vi "Read Full Output.vi"(6 "maximal byte count (-1)":i32=-1, 7 "timeout [ms]":u32=10, 8 "error in":errorcluster, 11 "GOLPI ref. in":T1={"pipe handle"={"lv_proc.dll file path"=path "", "process instance handle"=[], "debug mode"=FALSE, "debug data"=[]}, "fast read timeout [ms]"=500, "fast read settle time [ms]"=10, "fast read to multiple [ms]"=1, "max elements per input line"=100, "slow read timeout [ms]"=5000, "stdin double format specifier"="%_16e", "max elements per stdout output column"=100, "console mode bitstream"=FALSE, "bitstream first read timeout [ms]"=1000, "bitstream read timeout [ms]"=50, "struct transfer possible"=FALSE, "matlab mode"=FALSE}) -> (0 "error out":errorcluster, 2 "read buffer":string, 3 "GOLPI ref. out":T1={"pipe handle"={"lv_proc.dll file path"=path "", "process instance handle"=[], "debug mode"=FALSE, "debug data"=[]}, "fast read timeout [ms]"=500, "fast read settle time [ms]"=10, "fast read to multiple [ms]"=1, "max elements per input line"=100, "slow read timeout [ms]"=5000, "stdin double format specifier"="%_16e", "max elements per stdout output column"=100, "console mode bitstream"=FALSE, "bitstream first read timeout [ms]"=1000, "bitstream read timeout [ms]"=50, "struct transfer possible"=FALSE, "matlab mode"=FALSE}, 5 "bytes remaining":i32)   [LabVIEW 2020, in "GOLPI library.lvlib"]
doc: "Reads full output of GNU Octave in stdout pipe.\nIf timeout is exceeded (i.e. buffer contains too many characters), returns only part of buffer and returns number of bytes remaining in the stdout (if any).\nReading also stops if maximal byte count terminal is set to natural nonzero value and number of red bytes reaches this limit.\n\n---\nGOLPI works only with lv_proc.dll library, which is part of vipm package or should be delivered together with packed library. Placement of this dll is selected in terminal of Start GNU Octave.vi."
uses:
  GOLPI library.lvlib
  GOLPI reference Type Def.ctl
  Pipe Handle.ctl
  Custom Error Codes Enum Type Def.vi
  LV Process library.lvlib
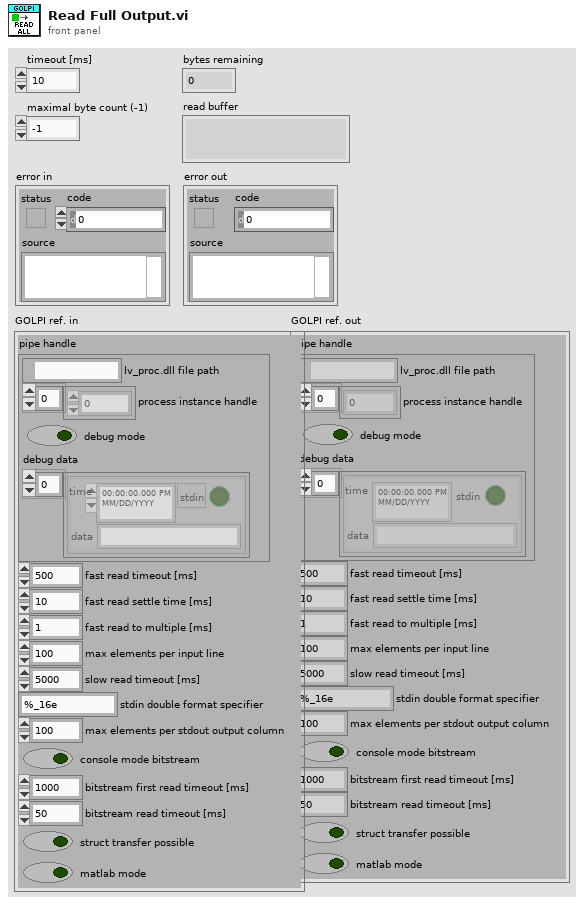
[diagram p1: front panel]
types:
  T1 = typedef "GOLPI library.lvlib/GOLPI reference Type Def.ctl" = cluster{"pipe handle":T2, "fast read timeout [ms]":u32, "fast read settle time [ms]":u32, "fast read to multiple [ms]":u32, "max elements per input line":u32, "slow read timeout [ms]":u32, "stdin double format specifier":string, "max elements per stdout output column":u32, "console mode bitstream":bool, "bitstream first read timeout [ms]":u32, "bitstream read timeout [ms]":u32, "struct transfer possible":bool, "matlab mode":bool}
  T2 = typedef "LV Process library.lvlib/Pipe Handle.ctl" = cluster{"lv_proc.dll file path":path, "process instance handle":u32[], "debug mode":bool, "debug data":cluster{"time":timestamp, "stdin":bool, "data":string}[]}
  T3 = typedef "GOLPI library.lvlib/Custom Error Codes Enum Type Def.vi" = enum16{"no error", "00 working directory PAR1 missing", "01 octave binary PAR1 missing", "02 octave report error PAR1", "03 empty output last cmd PAR1", "04 missing temporary file PAR1", "05 pwd PAR 1 not exist", "06 oct package not installed", "07 octave default binary missing", "10 var PAR1 not string, vect", "11 var PAR1 not num, scal, ~compl", "12 var PAR1 not num, scal, compl", "13 var PAR1 not num, vect, ~compl", "14 var PAR1 not num, vect, compl", "15 var PAR1 not num, mat, ~compl", "16 var PAR1 not num, mat, ~compl", "30 read timeout", "60 bitstream transport failed", "61 bitstream decode error PAR1", "62 bitstream cannot be set", "70 struct transfer not possible", "80 struct: cluster elem. PAR1 not implem.", "81 struct: structure field PAR1 not implem.", "82 struct: size mismatch of PAR1", "83 struct: type mismatch of PAR1", "98 internal error", "99 not finished", "90 Not supported in Matlab mode", "91 Matlab variable transfer error", "92 Matlab Script Error"}
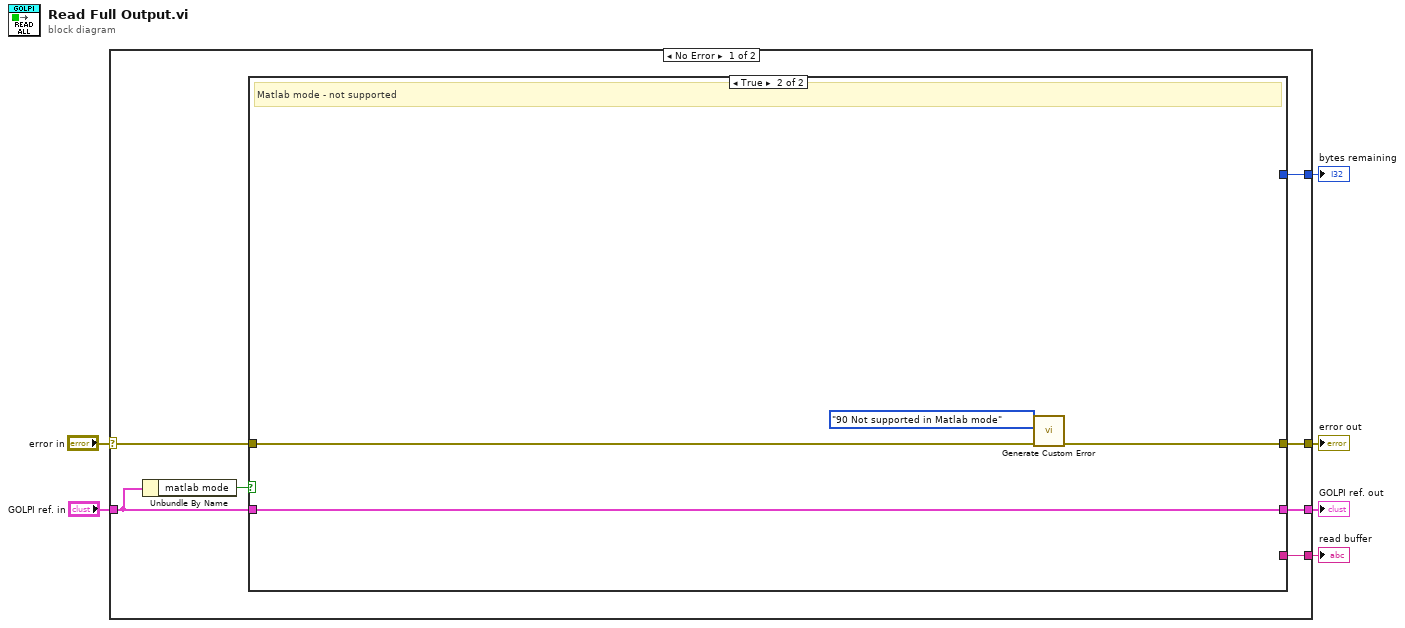
[diagram p0: block diagram]
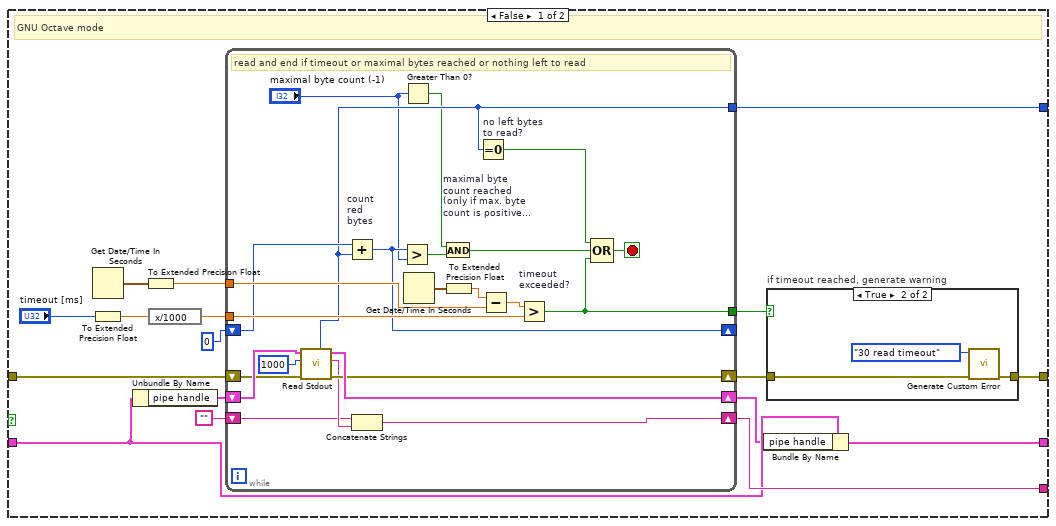
[diagram p2: hidden frame]
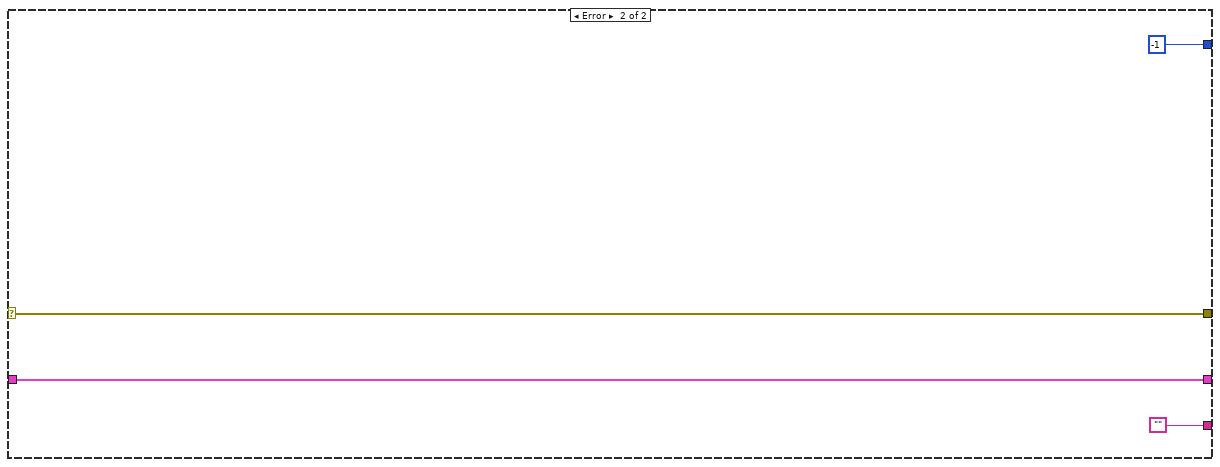
[diagram p4: hidden frame]
diagram:
  n1 = case shown="No Error" "error in" {
    selector: "error in" -> [w9 w62]
    tunnel: [w13 ""] -> w6
    tunnel: [w12 -1 ("bytes remaining")] -> w5
    tunnel: "GOLPI ref. in" -> [w8 w65]
    tunnel: [w11 w65] -> w3
    tunnel: [w10 w62] -> w2
    frame No Error {
      n2 = Unbundle By Name(w8) -> ("matlab mode"=w7:bool)
      n3 = case shown="True" w7 {
        tunnel: [w30 _] -> w13
        tunnel: [w29 _] -> w12
        tunnel: w8 -> [w26 w61]
        tunnel: [w25 w61] -> w11
        tunnel: [w22 w59] -> w10
        tunnel: w9 -> [w19 w60]
        frame False {
          # "GNU Octave mode"
          n4 = Get Date/Time In Seconds() -> (seconds since 1Jan1904=w18:timestamp)
          n5 = To Extended Precision Float(1:"timeout [ms]") -> (0:w16:ext)
          n6 = Unbundle By Name(w26) -> ("pipe handle"=w24:T2)
          n7 = To Extended Precision Float(1:w18) -> (0:w17:ext)
          n8 = expression code="x/1000"(w16) -> (w14:ext)
          n9 = while {
            tunnel: [w43] -> w29
            shift-right: [w56] -> w23
            shift-left: w24 -> [w57]
            shift-right: [w51] -> w30
            shift-left: "" -> [w52]
            tunnel: w17 -> [w50]
            tunnel: w14 -> [w47]
            shift-right: [w42] -> _
            shift-left: 0 -> [w45]
            shift-right: [w55] -> w21
            shift-left: w19 -> [w54]
            tunnel: [w37] -> w20
            stop <- w46 stop-if-true
            # "read and end if timeout or maximal bytes reached or nothing left to read"
            n10 = call "Read Stdout.vi"("error in"=w54, "byte count"=1000, "pipe in"=w57) -> ("error out"=w55:errorcluster, "read buffer"=w53:string, "pipe out"=w56:T2, "bytes remaining"=w43:i32)  [unwired: 3 in, 2 out]
            n11 = Add "count\nred\nbytes"(x=w45, y=w43) -> (x+y=w42:i32)
            n12 = Concatenate Strings(w52, w53) -> (w51:string)
            n13 = Greater?(x=w42, y="maximal byte count (-1)") -> (0:w39:bool)
            n14 = Greater Than 0?(x="maximal byte count (-1)") -> (x > 0?=w41:bool)
            n15 = Get Date/Time In Seconds() -> (seconds since 1Jan1904=w36:timestamp)
            n16 = And "maximal byte\ncount reached\n(only if max. byte\ncount is positive\nand nonzero)?"(x=w41, y=w39) -> (x .and. y?=w38:bool)
            n17 = To Extended Precision Float(1:w36) -> (0:w35:ext)
            n18 = Equal To 0? "no left bytes\nto read?"(x=w43) -> (x = 0?=w48:bool)
            n19 = Subtract(x=w35, y=w50) -> (x-y=w49:ext)
            n20 = Greater? "timeout\nexceeded?"(x=w49, y=w47) -> (0:w37:bool)
            n21 = Compound Arithmetic op=OR(w48, w38, w37) -> (w46:bool)
          }
          n22 = Bundle By Name(cluster=w26, "pipe handle"=w23) -> (w25:T1)
          n23 = case "if timeout reached, generate warning" shown="True" w20 {
            tunnel: [w31 w32] -> w22
            tunnel: w21 -> [w31 w33]
            frame False {
            }
            frame True {
              n24 = call "Generate Custom Error.vi"("error in"=w33, "GOLPI error"=Custom_Error_Codes_Enum_Type_Def.vi."30 read timeout") -> ("error out"=w32:errorcluster)  [unwired: 9 in]
            }
          }
        }
        frame True {
          # "Matlab mode - not supported"
          n25 = call "Generate Custom Error.vi"("error in"=w60, "GOLPI error"=Custom_Error_Codes_Enum_Type_Def.vi."90 Not supported in Matlab mode") -> ("error out"=w59:errorcluster)  [unwired: 9 in]
        }
      }
    }
    frame Error {
    }
  }
  "error out" <- w2
  "read buffer" <- w6
  "bytes remaining" <- w5
  "GOLPI ref. out" <- w3
